vi "Test Class Control Panel.vi"(8 "error in (no error)":errorcluster, 11 "Class":refnum<class "Test Class.lvclass">) -> (0 "error out":errorcluster, 3 "Test Class out":refnum<class "Test Class.lvclass">)   [LabVIEW 2015, in "Test Class.lvclass"]
uses:
  Test Class.lvclass
  Test FP data.ctl
panel:
  in  "Data":T1={"Channels to scan"=[], "Scan settling, s"=10.0, "Read temperature"=TRUE, "Read heater"=FALSE, "Control Instrument"=FALSE, "Set point"=0.0, "Heater Range"=enum."Off", "Test"=0.0}
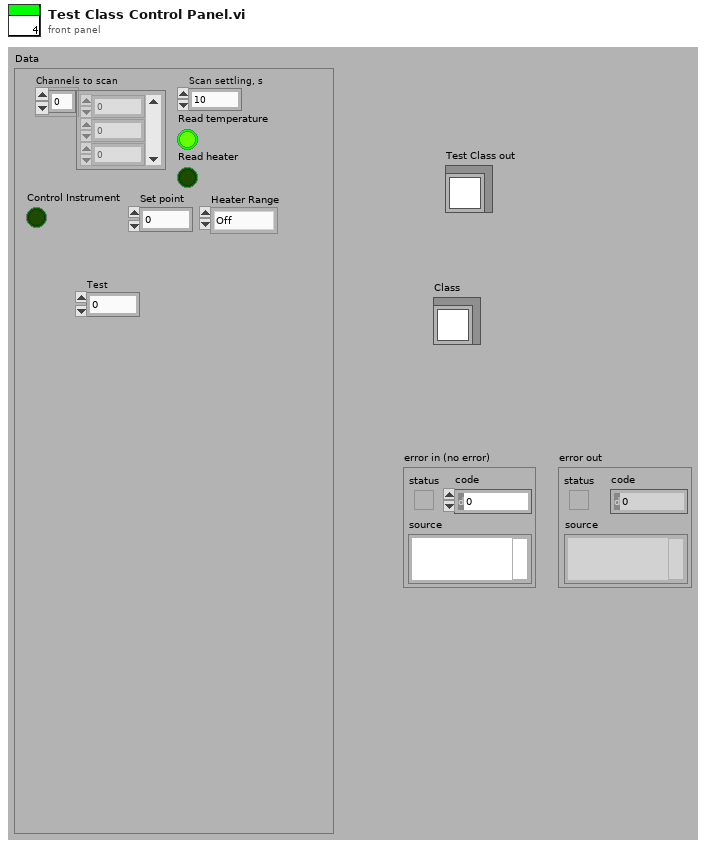
[diagram p1: front panel]
types:
  T1 = typedef "Test FP data.ctl" = cluster{"Channels to scan":i32[], "Scan settling, s":dbl, "Read temperature":bool, "Read heater":bool, "Control Instrument":bool, "Set point":dbl, "Heater Range":enum16{"Off", "31.6uA", "100uA", "316uA", "1mA", "3.16uA", "31.6mA", "100mA", "10mA"}, "Test":dbl}
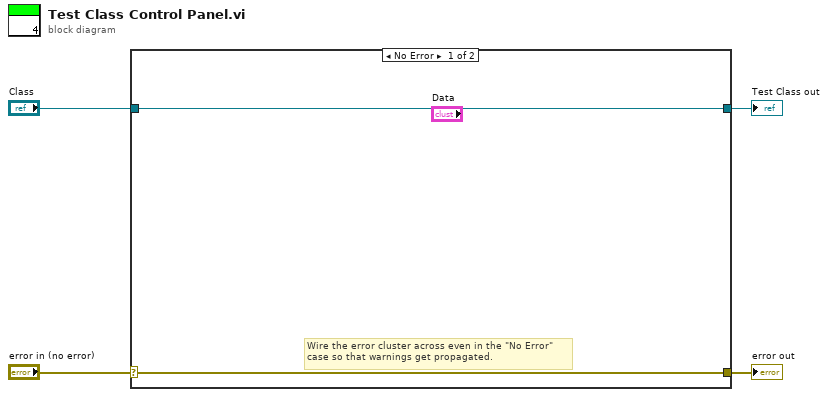
[diagram p0: block diagram]
diagram:
  n1 = case shown="No Error" "error in (no error)" {
    selector: "error in (no error)" -> [w5 w8]
    tunnel: [w5 w8] -> w3
    tunnel: [w6 w7] -> w1
    tunnel: "Class" -> [w6 w7]
    frame No Error {
      # "Wire the error cluster across even in the \"No Error\"\ncase so that warnings get propagated."
    }
    frame Error {
    }
  }
  "error out" <- w3
  "Test Class out" <- w1
